vi "WPI_CameraGet Image From HTTP Controller.vi"(4 "Camera Settings":T2={"name"="", "fps"=30, "compression"=30, "Image Size"=enum."320x240"}, 6 "Unflatten":bool, 8 "error in (no error)":errorcluster, 9 "Close?":bool, 10 "Controller Address":string, 11 "Image":T3) -> (0 "error out":errorcluster, 2 "Bandwidth (Mbps)":dbl=30.0, 3 "Image Out":T3(plugin-control))   [LabVIEW 2017]
doc: "Retrieves a specific image from the image data that the camera connected to the CompactRIO device you specify acquired. Use this VI in the FRC dashboard project on the host computer.\n\nThis software is licensed. Open the labview\\readme\\WPI Robotics Library Open Source License.txt file for more information."
uses:
  <vilib>/vision/Image Controls.llb/IMAQ Image.ctl
  <vilib>/Rock Robotics/WPI/Camera/WPI_CameraImageSize.ctl
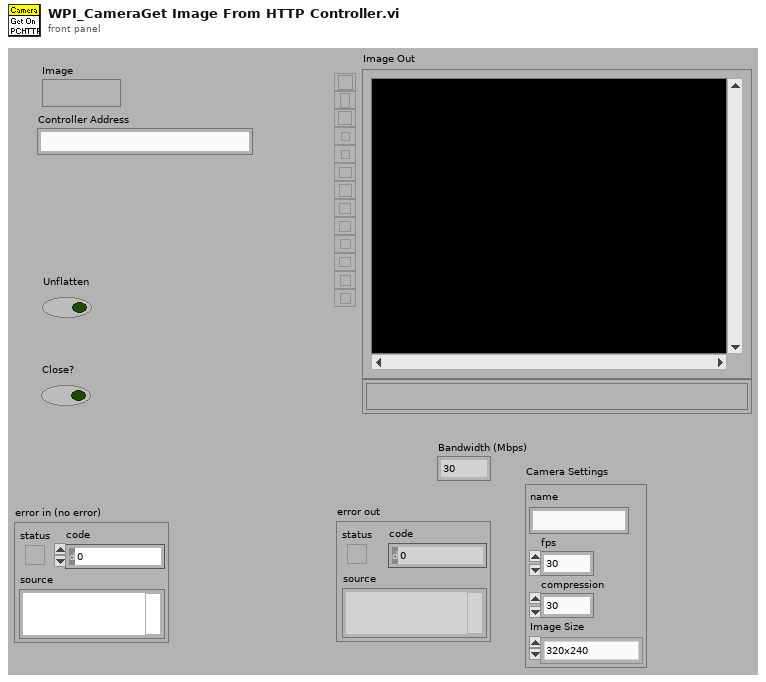
[diagram p1: front panel]
types:
  T1 = typedef "WPI_CameraImageSize.ctl" = enum16{"640x480", "320x240", "160x120", "Custom"}
  T2 = cluster{"name":string, "fps":i32, "compression":i32, "Image Size":T1}
  T3 = typedef "IMAQ Image.ctl" = refnum<image>
  T4 = cluster{"Camera Name":string, "Size":string, "Frame Rate":i32, "Compression":i32}
  T5 = cluster{"name":bool, "fps":bool, "compression":bool, "Image Size":bool}
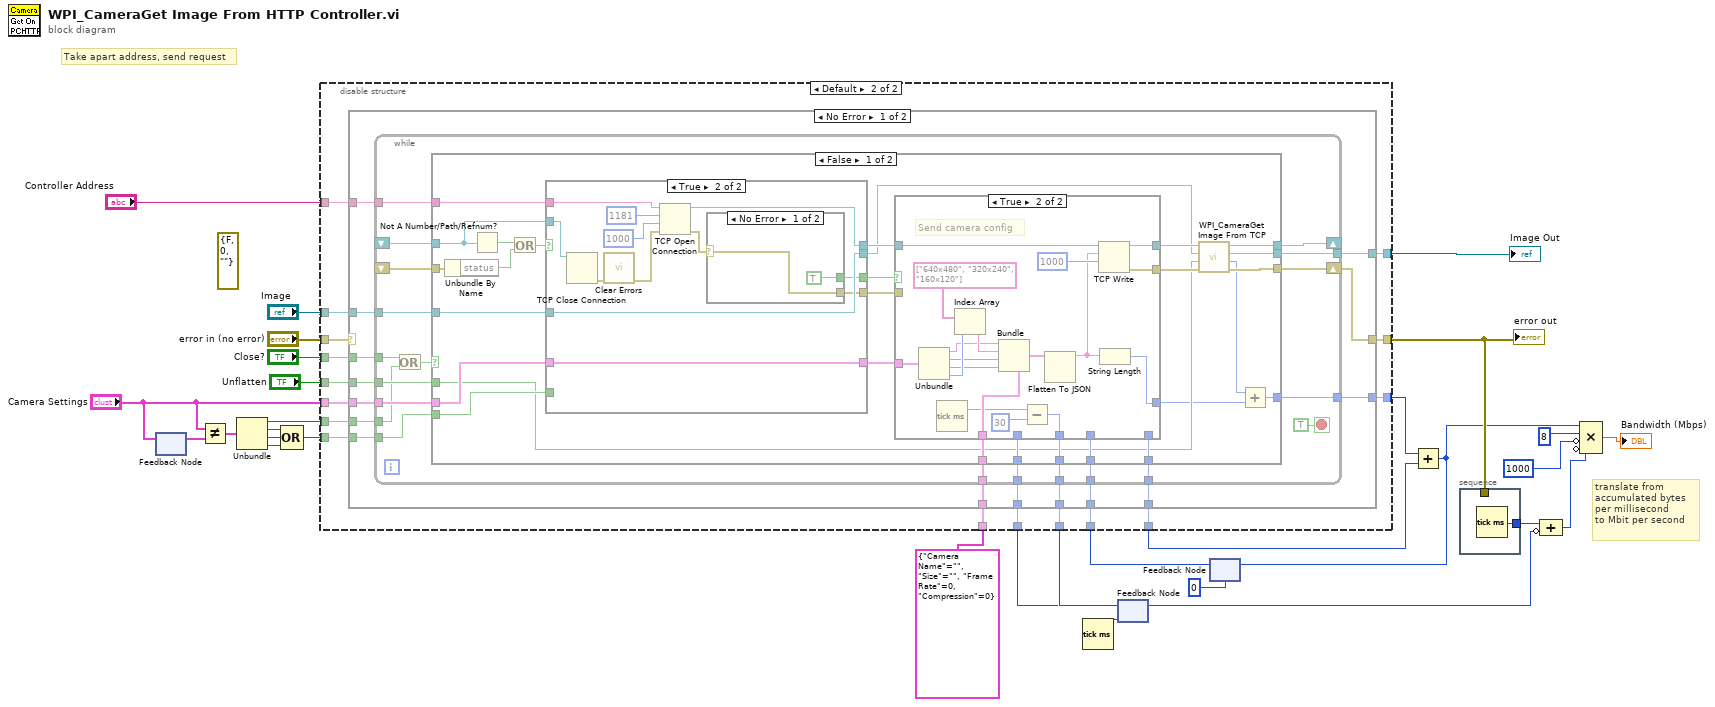
[diagram p0: block diagram]
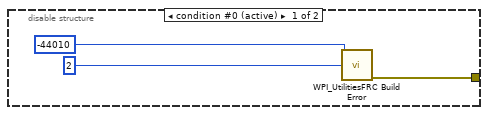
[diagram p2: hidden frame]
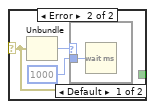
[diagram p5: hidden frame]
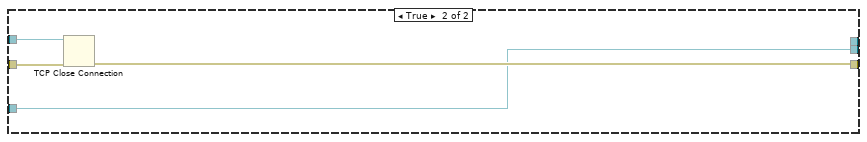
[diagram p7: hidden frame]
diagram:
  (unwired) errorcluster {"status"=FALSE, "code"=0, "source"=""} ("error constant")
  # "Take apart address, send request"
  # "translate from\naccumulated bytes\nper millisecond \nto Mbit per second"
  n1 = feedback-in #1("Camera Settings") -> ()
  n2 = feedback #1() -> (w23:T2)  [unwired: 1 in]
  n3 = Not Equal?(x="Camera Settings", y=w23) -> (x != y?=w5:T5)
  n4 = Unbundle(w5) -> ("name"=w6:bool, "fps"=w2:bool, "compression"=w3:bool, "Image Size"=w4:bool)
  n5 = Compound Arithmetic op=OR(w2, w3, w4) -> (w1:bool)
  n6 = Tick Count (ms)() -> (millisecond timer value=w22:u32)
  n7 = feedback #2(w22) -> (w12:u32)
  n8 = feedback #3(0) -> (w11:i32)
  n9 = disable-structure shown="Default" {
    disable-tunnel: "error in (no error)" -> [_ w48]
    disable-tunnel: [w30 w47] -> w15
    disable-tunnel: "Close?" -> [_ w46]
    disable-tunnel: "Image" -> [_ w45]
    disable-tunnel: [_ w44] -> w26
    disable-tunnel: "Controller Address" -> [_ w43]
    disable-tunnel: "Unflatten" -> [_ w42]
    disable-tunnel: "Camera Settings" -> [_ w41]
    disable-tunnel: w6 -> [_ w40]
    disable-tunnel: [_ w39] -> w13
    disable-tunnel: w12 -> [_ w38]
    disable-tunnel: w11 -> [_ w37]
    disable-tunnel: [_ w36] -> w10
    disable-tunnel: [_ w35] -> w9
    disable-tunnel: T4 {"Camera Name"="", "Size"="", "Frame Rate"=0, "Compression"=0} ("cluster") -> [_ w34]
    disable-tunnel: w1 -> [_ w33]
    frame condition #0 (active) {
      n10 = call <vilib>:"WPI_UtilitiesFRC Build Error.vi"("error code"=-44010 ("code"), "chain levels to remove (1)"=2) -> ("error out"=w30:errorcluster)  [unwired: 3 in, 10 out]
    }
    frame condition #1 {
      n11 = case shown="No Error" w48 {
        selector: w48 -> [_ w163]
        tunnel: [w63 w163] -> w47
        tunnel: w46 -> [w62 _]
        tunnel: w45 -> [w61 w162]
        tunnel: [w60 w162] -> w44
        tunnel: w43 -> [w59 _]
        tunnel: w42 -> [w58 _]
        tunnel: w41 -> [w57 _]
        tunnel: w40 -> [w56 _]
        tunnel: [w55 w161] -> w39
        tunnel: w38 -> [w54 w161]
        tunnel: w37 -> [w53 w160]
        tunnel: [w52 w160] -> w36
        tunnel: [w51 _] -> w35
        tunnel: w34 -> [w50 _]
        tunnel: w33 -> [w49 _]
        frame No Error {
          n12 = while {
            shift-right: [w83] -> w63
            shift-left: _ -> [w81]
            shift-right: [w82] -> _
            shift-left: _ -> [w80]
            tunnel: w62 -> [w73]
            tunnel: w61 -> [w78]
            tunnel: [w77] -> w60
            tunnel: w59 -> [w76]
            tunnel: w58 -> [w75]
            tunnel: w57 -> [w74]
            tunnel: w56 -> [w71]
            tunnel: [w67] -> w55
            tunnel: w54 -> [w64]
            tunnel: w53 -> [w66]
            tunnel: [w65] -> w52
            tunnel: [w70] -> w51
            tunnel: w50 -> [w69]
            tunnel: w49 -> [w68]
            stop <- TRUE stop-if-true
            n13 = Or(x=w73, y=w71) -> (x .or. y?=w72:bool)
            n14 = case shown="False" w72 {
              tunnel: [w88 w157] -> w83
              tunnel: [w90 _] -> w82
              tunnel: w81 -> [w111 w158]
              tunnel: w80 -> [w108 w159]
              tunnel: w78 -> [w107 w156]
              tunnel: [w91 w156] -> w77
              tunnel: w76 -> [w106 _]
              tunnel: w75 -> [w87 _]
              tunnel: w74 -> [w105 _]
              tunnel: [w84 _] -> w70
              tunnel: w69 -> [w102 _]
              tunnel: w68 -> [w100 _]
              tunnel: [w99 _] -> w67
              tunnel: w66 -> [w98 _]
              tunnel: [w97 _] -> w65
              tunnel: w64 -> [w96 _]
              frame False {
                n15 = Unbundle By Name(w111) -> ("status"=w104:bool)
                n16 = Not A Number/Path/Refnum?(number/path/refnum=w108) -> (NaN/Path/Refnum?=w110:bool)
                n17 = Or(x=w110, y=w104) -> (x .or. y?=w109:bool)
                n18 = case shown="True" w109 {
                  tunnel: [_ w139] -> w94
                  tunnel: [w134 w142] -> w95
                  tunnel: w108 -> [w134 w149]
                  tunnel: w107 -> [w135 w145]
                  tunnel: [w135 w145] -> w92
                  tunnel: w106 -> [_ w144]
                  tunnel: w105 -> [w137 w141]
                  tunnel: [w137 w141] -> w103
                  tunnel: [w136 w138] -> w101
                  tunnel: w100 -> [w136 _]
                  frame False {
                  }
                  frame True {
                    n19 = TCP Close Connection(connection ID=w149) -> (error out=w148:errorcluster)  [unwired: 1 in, 2 out]
                    n20 = call <vilib>:"Clear Errors.vi"("error in (no error)"=w148) -> ("error out"=w147:errorcluster)  [unwired: 1 in, 5 out]
                    n21 = TCP Open Connection(address=w144, remote port or service name=u16 1181 ("port"), timeout ms (60000)=1000 ("timeout ms (wait forever: -1)"), error in (no error)=w147) -> (connection ID=w142:refnum<k5>, error out=w140:errorcluster)  [unwired: 1 out]
                    n22 = case shown="No Error" w140 {
                      selector: w140 -> [w151 w153]
                      tunnel: [w151 w153] -> w139
                      tunnel: [TRUE _] -> w138
                      frame No Error {
                      }
                      frame Error {
                        n23 = Unbundle(w153) -> ("code"=w154:i32)  [unwired: 2 out]
                        n24 = case shown="Default" w154 {
                          tunnel: u32 1000 ("milliseconds to wait") -> [w155 _]
                          frame Default {
                            n25 = Wait (ms)(milliseconds to wait=w155) -> ()  [unwired: 1 out]
                          }
                          frame 56 {
                          }
                        }
                      }
                    }
                  }
                }
                n26 = case shown="True" w101 {
                  tunnel: w95 -> [w115 w133]
                  tunnel: [w115 w131] -> w93
                  tunnel: [w114 w130] -> w89
                  tunnel: w103 -> [_ w126]
                  tunnel: w102 -> [_ w128]
                  tunnel: [_ w119] -> w85
                  tunnel: w94 -> [w114 _]
                  tunnel: [w113 w118] -> w99
                  tunnel: w98 -> [w112 _]
                  tunnel: [w112 _] -> w97
                  tunnel: w96 -> [w113 _]
                  frame False {
                  }
                  frame True {
                    # "Send camera config"
                    n27 = Unbundle(w126) -> ("name"=w122:string, "fps"=w123:i32, "compression"=w124:i32, "Image Size"=w125:T1)
                    n28 = Tick Count (ms)() -> (millisecond timer value=w117:u32)
                    n29 = Index Array(array=string[] ["640x480", "320x240", "160x120"] ("Array"), index=w125) -> (element=w127:string)
                    n30 = Bundle(cluster=w128, "Camera Name"=w122, "Size"=w127, "Frame Rate"=w123, "Compression"=w124) -> (w129:T4)
                    n31 = Subtract(x=w117, y=30 ("timeout ms (25000)")) -> (x-y=w118:u32)
                    n32 = Flatten To JSON(anything=w129) -> (JSON string=w121:string)  [unwired: 2 in, 1 out]
                    n33 = TCP Write(connection ID=w133, data in=w121, 9:1000 ("timeout ms (25000)")) -> (connection ID out=w131:refnum<k5>, error out=w130:errorcluster)  [unwired: 1 in, 1 out]
                    n34 = String Length(string=w121) -> (length=w119:i32)
                  }
                }
                n35 = call <vilib>:"WPI_CameraGet Image From TCP.vi"("error in (no error)"=w89, "Unflatten"=w87, "Image In"=w92, "connection ID"=w93) -> ("error out"=w88:errorcluster, "Size"=w86:i32, "Image Out"=w91:T3, "connection ID (dup)"=w90:refnum<k5>)  [unwired: 1 in, 3 out]
                n36 = Add(x=w86, y=w85) -> (x+y=w84:i32)
              }
              frame True {
                n37 = TCP Close Connection(connection ID=w159, error in (no error)=w158) -> (error out=w157:errorcluster)  [unwired: 2 out]
              }
            }
          }
        }
        frame Error {
        }
      }
    }
  }
  "error out" <- w15
  "Image Out" <- w26
  n38 = feedback-in #2(w13) -> ()
  n39 = Add(x=w9, y=w10) -> (x+y=w14:i32)
  n40 = feedback-in #3(w14) -> ()
  n41 = stacked-sequence {
    tunnel: [w164] -> w18
    tunnel: w15 -> [_]
    frame #0 {
      n42 = Tick Count (ms)() -> (millisecond timer value=w164:u32)
    }
  }
  n43 = Compound Arithmetic op=ADD(w18, invert w13) -> (w19:u32)
  n44 = Compound Arithmetic op=MULTIPLY(w14, 8 ("timeout ms (25000)"), invert 1000 ("timeout ms (25000)"), invert w19) -> (→"Bandwidth (Mbps)":dbl)
